vi "Global PCAN Baudrate.vi"() -> ()   [LabVIEW 2020]
uses:
  source/PCAN Baud.ctl
  source/PCANBasic.lvlib
panel:
  in  "PCAN Baudrate":T1=81 items=["PCAN_BAUD_1M"=20, "PCAN_BAUD_800K"=22, "PCAN_BAUD_500K"=28, "PCAN_BAUD_250K"=284, "PCAN_BAUD_125K"=796, "PCAN_BAUD_100K"=17199, "PCAN_BAUD_95K"=49998, "PCAN_BAUD_83K"=34091, "PCAN_BAUD_50K"=18223, "PCAN_BAUD_47K"=5140, "PCAN_BAUD_33K"=35631, "PCAN_BAUD_20K"=21295, "PCAN_BAUD_10K"=26415, "PCAN_BAUD_5K"=32639]
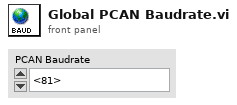
[diagram p1: front panel]
types:
  T1 = typedef "PCANBasic.lvlib/PCAN Baud.ctl" = u16
diagram:
